vi "DVR Reader.vi"(0 "Get Value":bool, 5 "Stop":bool, 11 "Error In":errorcluster) -> (4 "Numeric Output":dbl, 15 "Error Out":errorcluster)   [LabVIEW 2023]
doc: "This VI reads the reference of the DVR and has a getvalue button which when pressed will display the current value in the DVR in numeric output."
uses:
  Controls/Operation.ctl
panel:
  # "Instructions:\n1. Run the VI.\n2. Click Get Value to display the output in the indicator.\n3.  Press Stop button or panel close to stop the VI."
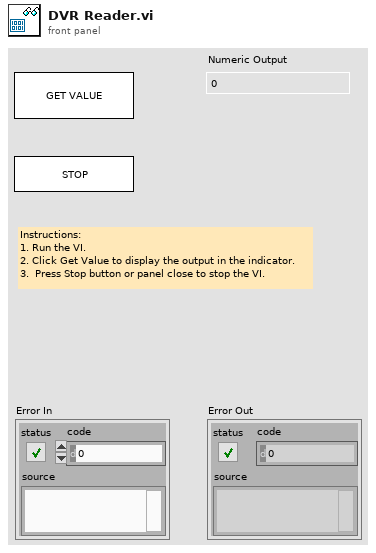
[diagram p1: front panel]
types:
  T1 = typedef "Operation.ctl" = enum16{"Write Ref", "Read Ref"}
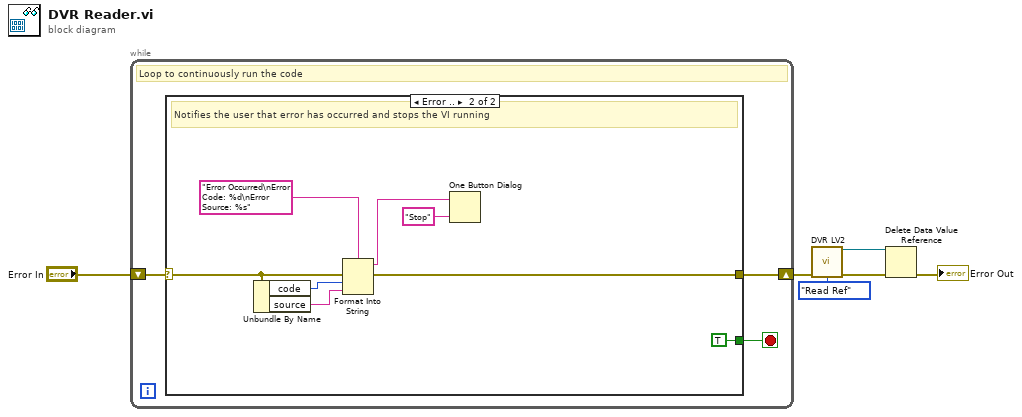
[diagram p0: block diagram]
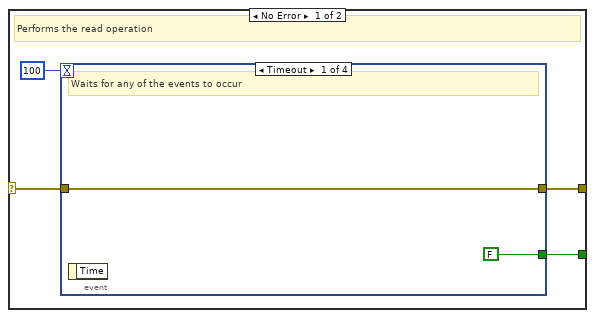
[diagram p2: hidden frame]
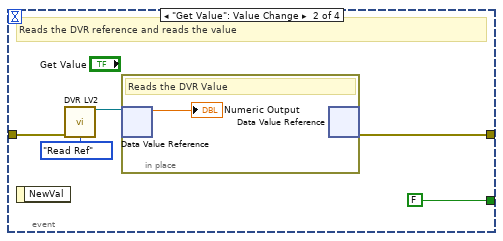
[diagram p3: hidden frame]
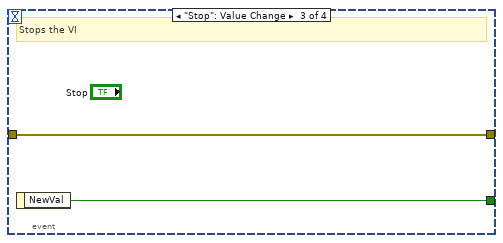
[diagram p4: hidden frame]
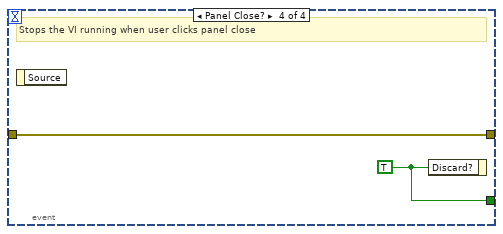
[diagram p5: hidden frame]
diagram:
  n1 = while {
    shift-right: [w8] -> w6
    shift-left: "Error In" -> [w7]
    stop <- w9 stop-if-true
    # "Loop to continuously run the code"
    n2 = case shown="Error .." w7 {
      selector: w7 -> [w10 w28]
      tunnel: [w13 TRUE ("Discard?")] -> w9
      tunnel: [w11 w31] -> w8
      frame No Error {
        # "Performs the read operation"
        n3 = event shown="[0] Timeout" {
          selector: _ -> [_ _ _ _]
          dyn-events: _ -> [_ _ _ _]
          timeout: 100 -> [_ _ _ _]
          tunnel: [FALSE ("NewVal") FALSE ("NewVal") w23 w25] -> w13
          tunnel: [w14 w19 w22 w24] -> w11
          tunnel: w10 -> [w14 w18 w22 w24]
          event Timeout {
            # "Waits for any of the events to occur"
            n4 = event-data() -> ()  [unwired: 1 in, 1 out]
          }
          event "Get Value": Value Change {
            # "Reads the DVR reference and reads the value"
            n5 = event-data() -> ()  [unwired: 1 in, 1 out]
            n6 = call "DVR LV2.vi"("error in (no error)"=w18, "Operation"=Operation."Read Ref") -> ("Data Value Refnum 2"=w17:refnum<data-value>)  [unwired: 12 in, 1 out]
            n7 = in-place {
              # "Reads the DVR Value"
              n8 = in-place-dvr #1(w17) -> (→"Numeric Output":dbl)  [unwired: 1 out]
              n9 = in-place-dvr #1() -> (w19:errorcluster)  [unwired: 1 in, 1 out]
            }
          }
          event "Stop": Value Change {
            # "Stops the VI"
            n10 = event-data() -> ("NewVal"=w23:bool)  [unwired: 1 in]
          }
          event Panel Close? {
            w25 = TRUE ("Discard?")
            # "Stops the VI running when user clicks panel close"
            n11 = event-data() -> ()  [unwired: 1 in, 1 out]
            n12 = event-data("Discard?"=w25) -> ()  [unwired: 1 in, 1 out]
          }
        }
      }
      frame Error {
        # "Notifies the user that error has occurred and stops the VI running"
        n13 = Unbundle By Name(w28) -> ("code"=w27:i32, "source"=w26:string)
        n14 = Format Into String(format string="Error Occurred\nError Code: %d\nError Source: %s" ("message"), error in=w28, w27, w26) -> (resulting string=w29:string, error out=w31:errorcluster)  [unwired: 1 in]
        n15 = One Button Dialog(message=w29, button name ("OK")="Stop") -> ()  [unwired: 1 out]
      }
    }
  }
  n16 = call "DVR LV2.vi"("error in (no error)"=w6, "Operation"=Operation."Read Ref") -> ("Data Value Refnum 2"=w2:refnum<data-value>, "error out"=w3:errorcluster)  [unwired: 12 in]
  n17 = Delete Data Value Reference(data value reference=w2, error in=w3) -> (error out=→"Error Out":errorcluster)  [unwired: 1 out]
